vi "simple_sequence_loop.vi"() -> ()   [LabVIEW 2021]
panel:
  out "Waveform Chart":dbl(graph)
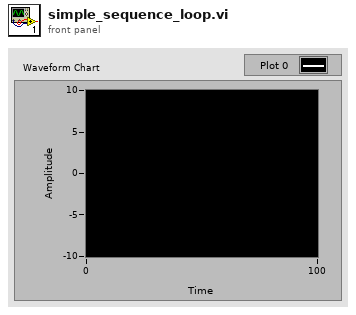
[diagram p1: front panel]
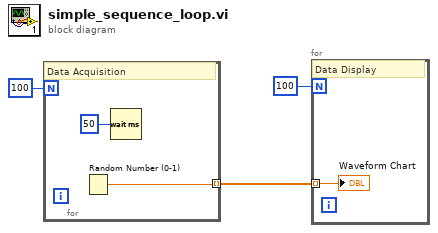
[diagram p0: block diagram]
diagram:
  n1 = for {
    N: 100 -> [_]
    tunnel: [w4] -> w1 mode=indexing
    # "Data Acquisition"
    n2 = Random Number (0-1)() -> (number: 0 to 1=w4:dbl)
    n3 = Wait (ms)(milliseconds to wait=u32 50) -> ()  [unwired: 1 out]
  }
  n4 = for {
    N: 100 -> [_]
    tunnel: w1 -> [w6] mode=indexing
    # "Data Display"
    "Waveform Chart" <- w6
  }
